vi "ex3-4.vi"() -> ()   [LabVIEW 2009]
panel:
  out "迴圈執行次數":i32
  out "X+Y":dbl
  in  "Y":dbl
  in  "X":dbl
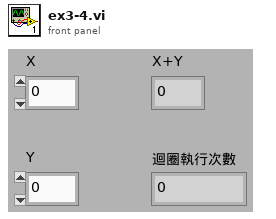
[diagram p1: front panel]
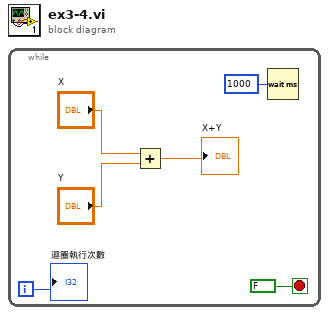
[diagram p0: block diagram]
diagram:
  n1 = while {
    i -> [w2]
    stop <- FALSE stop-if-true
    n2 = Add(x="X", y="Y") -> (x+y=→"X+Y":dbl)
    n3 = Wait (ms)(milliseconds to wait=u32 1000) -> ()  [unwired: 1 out]
    "迴圈執行次數" <- w2
  }
